vi "myRIO_BRig_Host_parse_uploadSettings.vi"() -> ()   [LabVIEW 2014]
panel:
  out "filedir":string
  out "filename":string
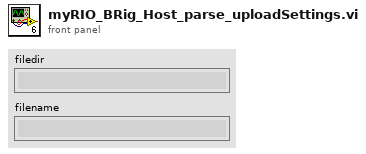
[diagram p1: front panel]
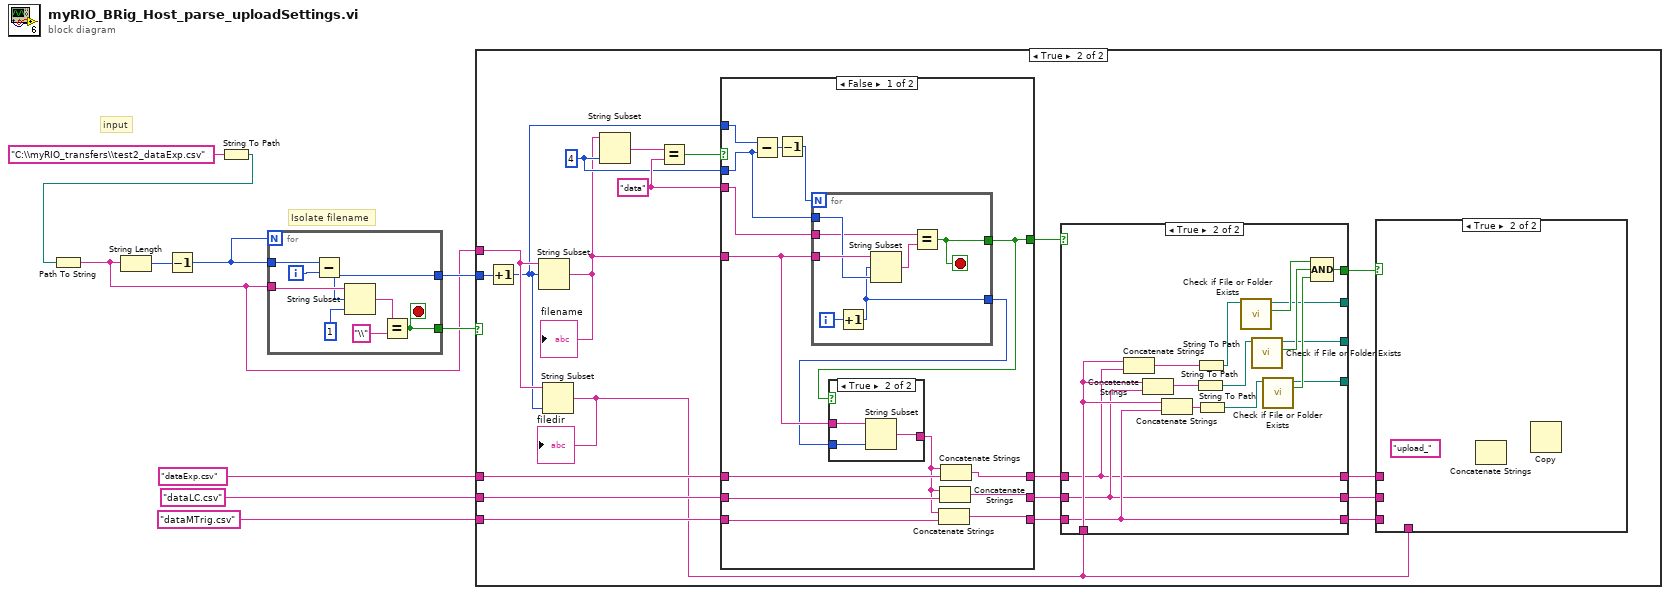
[diagram p0: block diagram]
diagram:
  # "Isolate filename"
  # "input"
  n1 = String To Path(string="C:\\myRIO_transfers\\test2_dataExp.csv") -> (path=w9:path)
  n2 = Path To String(path=w9) -> (string=w4:string)
  n3 = String Length(string=w4) -> (length=w8:i32)
  n4 = Decrement(x=w8) -> (x-1=w7:i32)
  n5 = for {
    N: w7 -> [_]
    tunnel: w7 -> [w16]
    tunnel: w4 -> [w14]
    tunnel: [w12] -> w5
    tunnel: [w11] -> w6
    i -> [w15]
    stop <- w11 stop-if-true
    n6 = Subtract(x=w16, y=w15) -> (x-y=w12:i32)
    n7 = String Subset(string=w14, offset (0)=w12, length (rest)=1 ("length (rest)")) -> (substring=w13:string)
    n8 = Equal?(x=w13, y="\\") -> (x = y?=w11:bool)
  }
  n9 = case shown="True" w6 {
    tunnel: w5 -> [_ w32]
    tunnel: w4 -> [_ w33]
    tunnel: "dataExp.csv" -> [_ w36]
    tunnel: "dataLC.csv" -> [_ w35]
    tunnel: "dataMTrig.csv" -> [_ w34]
    frame False {
    }
    frame True {
      w28 = "data" ("y")
      w27 = 4 ("length (rest)")
      n10 = Increment(x=w32) -> (x+1=w26:i32)
      n11 = String Subset(string=w33, offset (0)=w26) -> (substring=w25:string)  [unwired: 1 in]
      "filename" <- w25
      n12 = String Subset(string=w33, length (rest)=w26) -> (substring=w22:string)  [unwired: 1 in]
      "filedir" <- w22
      n13 = String Subset(string=w25, length (rest)=w27) -> (substring=w38:string)  [unwired: 1 in]
      n14 = Equal?(x=w38, y=w28) -> (x = y?=w37:bool)
      n15 = case shown="False" w37 {
        selector: w37 -> [_ w81]
        tunnel: w36 -> [w62 w84]
        tunnel: w35 -> [w60 w83]
        tunnel: w34 -> [w58 w82]
        tunnel: [w61 w84] -> w31
        tunnel: [w59 w83] -> w30
        tunnel: [w56 w82] -> w29
        tunnel: w28 -> [w68 _]
        tunnel: w27 -> [w69 _]
        tunnel: w26 -> [w70 _]
        tunnel: w25 -> [w64 _]
        tunnel: [w65 w81] -> w24
        frame False {
          n16 = Subtract(x=w70, y=w69) -> (x-y=w67:i32)
          n17 = Decrement(x=w67) -> (x-1=w66:i32)
          n18 = for {
            N: w66 -> [_]
            tunnel: w69 -> [w78]
            tunnel: w68 -> [w76]
            tunnel: w64 -> [w80]
            tunnel: [w75] -> w65
            tunnel: [w74] -> w63
            i -> [w79]
            stop <- w75 stop-if-true
            n19 = Increment(x=w79) -> (x+1=w74:i32)
            n20 = String Subset(string=w80, offset (0)=w74, length (rest)=w78) -> (substring=w77:string)
            n21 = Equal?(x=w76, y=w77) -> (x = y?=w75:bool)
          }
          n22 = case shown="True" w65 {
            tunnel: w64 -> [_ w73]
            tunnel: w63 -> [_ w72]
            tunnel: [_ w71] -> w57
            frame False {
            }
            frame True {
              n23 = String Subset(string=w73, length (rest)=w72) -> (substring=w71:string)  [unwired: 1 in]
            }
          }
          n24 = Concatenate Strings(w57, w58) -> (w56:string)
          n25 = Concatenate Strings(w57, w60) -> (w59:string)
          n26 = Concatenate Strings(w57, w62) -> (w61:string)
        }
        frame True {
        }
      }
      n27 = case shown="True" w24 {
        tunnel: w22 -> [_ w49]
        tunnel: w31 -> [_ w39]
        tunnel: w30 -> [_ w40]
        tunnel: w29 -> [_ w41]
        tunnel: [_ w45] -> w23
        tunnel: [_ w44] -> _
        tunnel: [_ w43] -> _
        tunnel: [_ w42] -> _
        tunnel: [_ w41] -> w21
        tunnel: [_ w40] -> w20
        tunnel: [_ w39] -> w19
        frame False {
        }
        frame True {
          n28 = Concatenate Strings(w49, w39) -> (w50:string)
          n29 = Concatenate Strings(w49, w40) -> (w51:string)
          n30 = Concatenate Strings(w49, w41) -> (w52:string)
          n31 = String To Path(string=w51) -> (path=w54:path)
          n32 = String To Path(string=w50) -> (path=w53:path)
          n33 = String To Path(string=w52) -> (path=w55:path)
          n34 = call <vilib>:"Check if File or Folder Exists.vi"("path"=w53) -> ("file or folder exists?"=w46:bool, "dup path"=w42:path)  [unwired: 8 in, 1 out]
          n35 = call <vilib>:"Check if File or Folder Exists.vi"("path"=w54) -> ("file or folder exists?"=w47:bool, "dup path"=w43:path)  [unwired: 8 in, 1 out]
          n36 = call <vilib>:"Check if File or Folder Exists.vi"("path"=w55) -> ("file or folder exists?"=w48:bool, "dup path"=w44:path)  [unwired: 8 in, 1 out]
          n37 = Compound Arithmetic op=AND(w46, w47, w48) -> (w45:bool)
        }
      }
      n38 = case shown="True" w23 {
        tunnel: w22 -> [_ _]
        tunnel: w21 -> [_ _]
        tunnel: w20 -> [_ _]
        tunnel: w19 -> [_ _]
        frame False {
        }
        frame True {
          (unwired) "upload_"
          n39 = Concatenate Strings() -> ()  [unwired: 3 in, 1 out]
          n40 = Copy() -> ()  [unwired: 5 in, 3 out]
        }
      }
    }
  }
